vi "NISE.remote.Get Devices List.vi"(0 "SLSC Remote in":refnum<class "SLSC Interface.lvclass">, 11 "error in (no error)":errorcluster) -> (4 "SLSC Remote out":refnum<class "SLSC Interface.lvclass">, 8 "Sys.Devices":refnum<k21>[](array[refnum]), 15 "error out":errorcluster)   [LabVIEW 2016, in "SLSC Interface.lvclass"]
uses:
  SLSC Interface Class/SLSC Interface.lvclass
  SLSC Interface Class/SLSC Interface.lvclass/SLSC Interface.ctl
  SLSC Interface Class/NISE.Read client handle.vi
  SLSC Interface Class/NISE.Read URL.vi
  SLSC Interface Class/NISE.Read session.vi
  <vilib>/NI/NI JSONRPC Server Framework/Classes/Server/server.Format Client Request (Auto-Increment).vi
  <vilib>/httpClient/POSTBuffer.vi
  <vilib>/httpClient/LabVIEWHTTPClient.lvlib
  <vilib>/NI/NI JSONRPC Server Framework/Classes/Server/JSONRPC Server.lvclass
  <vilib>/NI/JSON Support for LabVIEW/JSON Value/JSON Value.lvclass
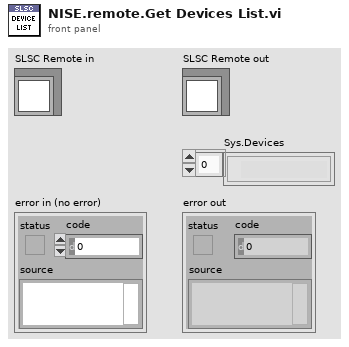
[diagram p1: front panel]
types:
  T1 = typedef "LabVIEWHTTPClient.lvlib/ClientHandle.ctl" = refnum<k1>
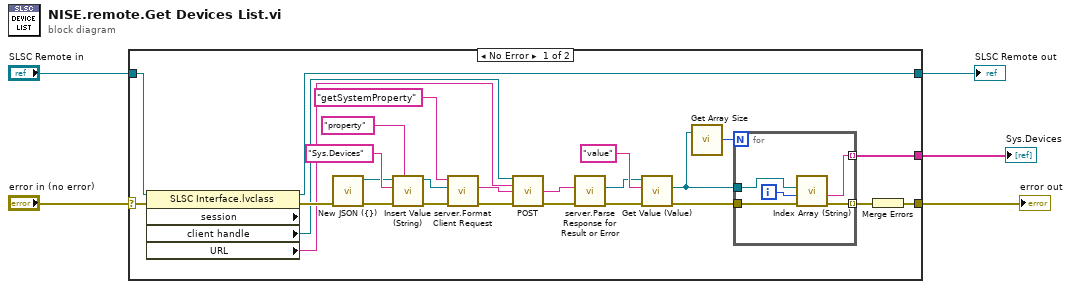
[diagram p0: block diagram]
diagram:
  n1 = case shown="No Error" "error in (no error)" {
    selector: "error in (no error)" -> [w29 w37]
    tunnel: "SLSC Remote in" -> [w31 w38]
    tunnel: [w30 w38] -> w3
    tunnel: [w9 w37] -> w1
    tunnel: [w8 _] -> w2
    frame No Error {
      n2 = property class="SLSC Interface.lvclass" props=["session", "client handle", "URL"](reference=w31, error in=w29) -> (reference out=w30:refnum<class "SLSC Interface.lvclass">, error out=w28:errorcluster, "client handle"=w24:T1, "URL"=w23:string)  [unwired: 1 out]
      n3 = call <vilib>:"New JSON ({}).vi"("error in (no error)"=w28) -> ("error out"=w27:errorcluster, "JSON Value out"=w14:refnum<class "JSON Value.lvclass">)  [unwired: 9 in]
      n4 = call <vilib>:"Insert Value (String).vi"("key"="property" ("Name"), "error in (no error)"=w27, "value"="Sys.Devices" ("String"), "JSON Value in"=w14) -> ("error out"=w18:errorcluster, "JSON Value out"=w19:refnum<class "JSON Value.lvclass">)  [unwired: 5 in, 1 out]
      n5 = call-poly <vilib>:"server.Format Client Request.vi"("error in (no error)"=w18, "JSON Value in"=w19, "method"="getSystemProperty") -> ("error out"=w22:errorcluster, "Request String"=w25:string)  [unwired: 7 in]
      n6 = call-poly <vilib>:"POST.vi"("client handle"=w24, "url"=w23, "buffer"=w25, "error in (no error)"=w22) -> ("body"=w21:string, "error out"=w20:errorcluster)  [unwired: 8 in, 2 out]
      n7 = call <vilib>:"server.Parse Response for Result or Error.vi"("error in"=w20, "Response String In"=w21) -> ("error out"=w13:errorcluster, "JSON Value out"=w6:refnum<class "JSON Value.lvclass">)  [unwired: 7 in, 1 out]
      n8 = call <vilib>:"Get Value (Value).vi"("error in (no error)"=w13, "key"="value" ("Parameter Name"), "JSON Value in"=w6) -> ("error out"=w11:errorcluster, "JSON Value out"=w7:refnum<class "JSON Value.lvclass">)  [unwired: 7 in]
      n9 = call <vilib>:"Get Array Size.vi"("JSON Value in"=w7) -> ("size(s)"=w12:i32)  [unwired: 1 in, 1 out]
      n10 = for {
        N: w12 -> [_]
        tunnel: w11 -> [w36]
        tunnel: [w35] -> w10 mode=indexing
        tunnel: [w34] -> w8 mode=indexing
        tunnel: w7 -> [w33]
        i -> [w32]
        n11 = call <vilib>:"Index Array (String).vi"("error in (no error)"=w36, "index"=w32, "JSON Value in"=w33) -> ("error out"=w35:errorcluster, "String"=w34:string)  [unwired: 7 in]
      }
      n12 = Merge Errors(w10) -> (w9:errorcluster)
    }
    frame Error {
    }
  }
  "error out" <- w1
  "SLSC Remote out" <- w3
  "Sys.Devices" <- w2
